vi "Configure BERT Pass Fail Criteria.vi"(7 "Pass Fail Criteria Threshold (0.01)":dbl=0.01, 8 "error in (no error)":errorcluster, 9 "Pass Fail Criteria Mode (0: Cycle End)":i32(ring) items=["Cycle End", "Fail Hold"], 10 "Enable Pass Fail Criteria (F: Disable)":bool, 11 "VISA resource name":refnum<visa-resource-name>) -> (0 "error out":errorcluster, 3 "VISA resource name out":refnum<visa-resource-name>)   [LabVIEW 2018, in "Agilent PSG MXG Series.lvlib"]
doc: "Configures the pass/fail judgment function for the comparator.\n\n<b>Note:</b>\nIt is applicable for N5172B/82B with <b>Option UN7</b> only."
uses:
  Agilent PSG MXG Series.lvlib
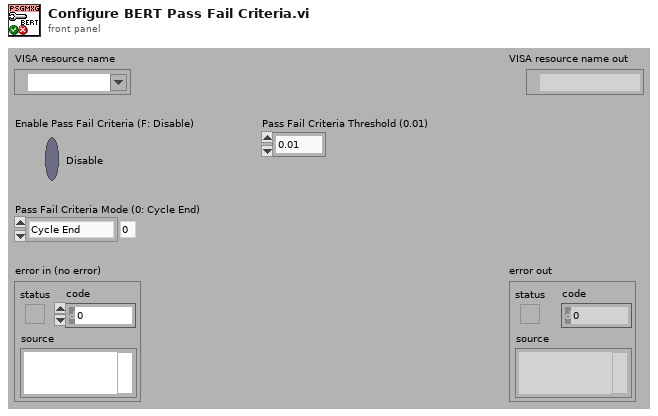
[diagram p1: front panel]
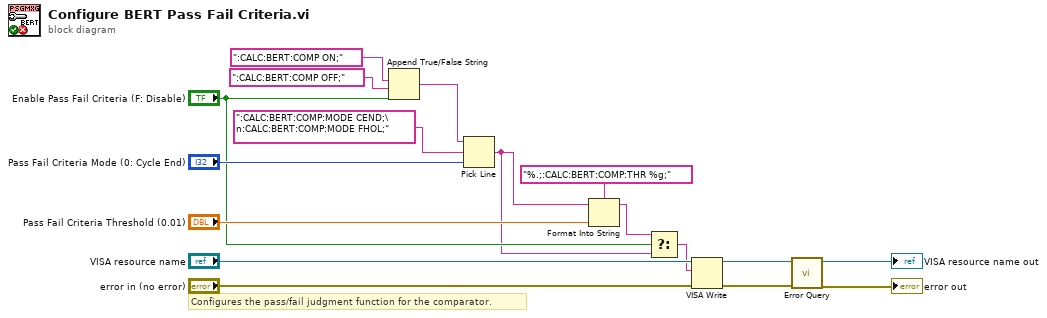
[diagram p0: block diagram]
diagram:
  # "Configures the pass/fail judgment function for the comparator."
  n1 = Append True/False String(1:"Enable Pass Fail Criteria (F: Disable)", 2:":CALC:BERT:COMP OFF;", 3:":CALC:BERT:COMP ON;") -> (0:w13:string)  [unwired: 1 in]
  n2 = Pick Line(string ("")=w13, multi-line string=":CALC:BERT:COMP:MODE CEND;\n:CALC:BERT:COMP:MODE FHOL;", line index="Pass Fail Criteria Mode (0: Cycle End)") -> (output string=w1:string)
  n3 = Format Into String(format string="%.;:CALC:BERT:COMP:THR %g;", initial string=w1, "Pass Fail Criteria Threshold (0.01)") -> (resulting string=w2:string)  [unwired: 1 in, 1 out]
  n4 = Select(t=w2, s="Enable Pass Fail Criteria (F: Disable)", f=w1) -> (s? t:f=w3:string)
  n5 = VISA Write(VISA resource name="VISA resource name", write buffer=w3, error in (no error)="error in (no error)") -> (VISA resource name out=w8:refnum<visa-resource-name>, error out=w7:errorcluster)  [unwired: 1 out]
  n6 = call "Error Query.vi"("error in (no error)"=w7, "VISA resource name"=w8) -> ("error out"=→"error out":errorcluster, "VISA resource name out"=→"VISA resource name out":refnum<visa-resource-name>)  [unwired: 6 in, 2 out]
